vi "Validate Checksum.vi"(10 "Response":string) -> (1 "Invalid Checksum?":bool, 2 "Remaining Response":string)   [LabVIEW 2015, in "Zaber A Series.lvlib"]
doc: "Expects a Zaber response string as an input. This VI inspects the response string to see if there is a checksum included. If not, then the same string is output and the boolean output is false. If there is a checksum, it is evaluated against the remainder of the response string. If the checksum is valid, the boolean output is false. If the checksum is not valid, the boolean output is true. Either way, the remainder of the response string (without the checksum) is output. The message start characters '/', '@', '#' and '!' are ignored and preserved if present. For more information on checksums, see the web page here: https://www.zaber.com/protocol-manual#topic_checksums."
uses:
  Zaber A Series.lvlib
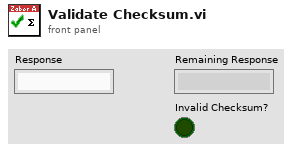
[diagram p1: front panel]
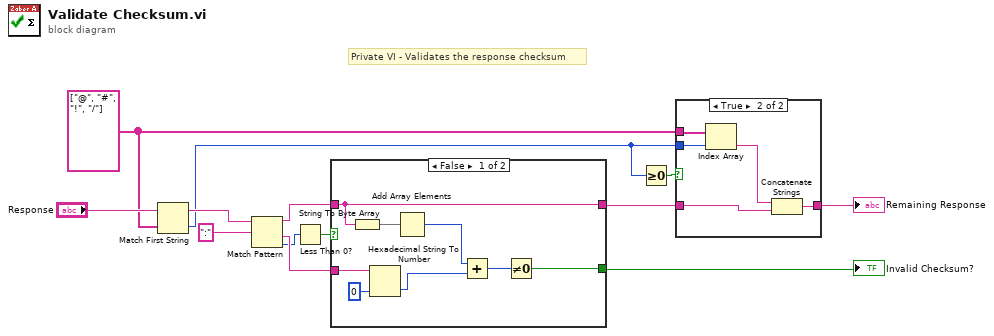
[diagram p0: block diagram]
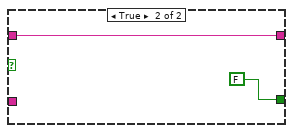
[diagram p3: hidden frame]
diagram:
  w2 = string[] ["@", "#", "!", "/"]
  # "Private VI - Validates the response checksum"
  n1 = Match First String(2:w2, 3:"Response") -> (0:w1:i32, 1:w6:string)
  n2 = Match Pattern(string=w6, regular expression=":") -> (before substring=w11:string, after substring=w12:string, offset past match=w9:i32)  [unwired: 1 in, 1 out]
  n3 = Less Than 0?(x=w9) -> (x < 0?=w10:bool)
  n4 = case shown="False" w10 {
    tunnel: w12 -> [w21 _]
    tunnel: w11 -> [w18 w23]
    tunnel: [w18 w23] -> w4
    tunnel: [w14 FALSE] -> w8
    frame False {
      n5 = String To Byte Array(string=w18) -> (unsigned byte array=w17:u8[])
      n6 = Hexadecimal String To Number(string=w21, default (0uL)=i8 0 ("default (0 U32)")) -> (number=w20:i8)  [unwired: 1 in, 1 out]
      n7 = Add Array Elements(numeric array=w17) -> (sum=w16:u8)
      n8 = Add(x=w16, y=w20) -> (x+y=w15:u8)
      n9 = Not Equal To 0?(x=w15) -> (x != 0?=w14:bool)
    }
    frame True {
    }
  }
  "Invalid Checksum?" <- w8
  n10 = Greater Or Equal To 0?(x=w1) -> (x >= 0?=w5:bool)
  n11 = case shown="True" w5 {
    tunnel: w4 -> [w24 w26]
    tunnel: [w24 w25] -> w3
    tunnel: w2 -> [_ w29]
    tunnel: w1 -> [_ w28]
    frame False {
    }
    frame True {
      n12 = Index Array(array=w29, index=w28) -> (element=w27:string)
      n13 = Concatenate Strings(w27, w26) -> (w25:string)
    }
  }
  "Remaining Response" <- w3
